vi "Find by Path Test.vi"() -> ()   [LabVIEW 2017]
uses:
  String Subset.vi
  Offset/Find Item Locations by Path.vi
  Parsing/Parse Full Path or Item Name.vi
  <vilib>/addons/_JKI Toolkits/Caraya/classes/Test/Test.lvclass
  <vilib>/addons/_JKI Toolkits/Caraya/classes/Assert/Assert.lvclass
  JSONtext.lvlib
panel:
  out "error out":errorcluster
  out "Path":string[](array[string])
  out "Time (s)":dbl[](array[numeric]) format="%#_3p"
  out "Array":string[](array[string])
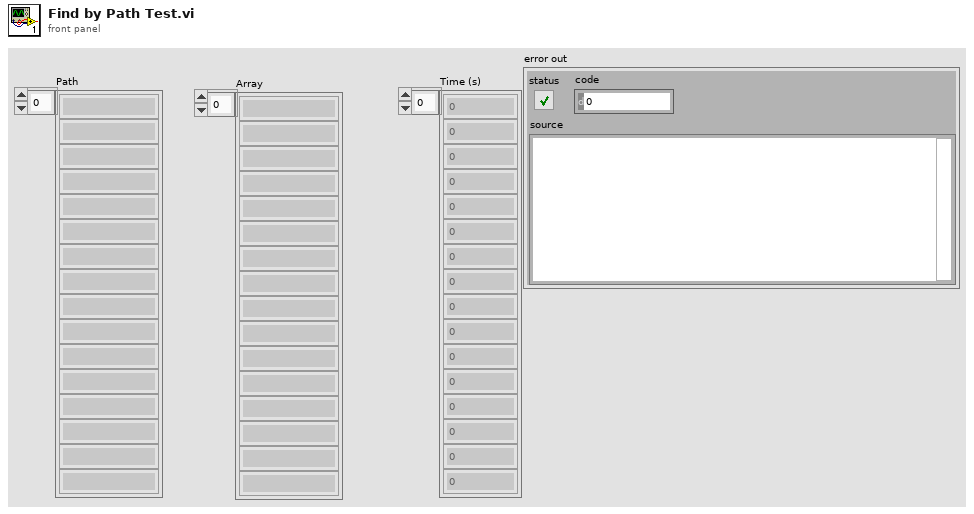
[diagram p1: front panel]
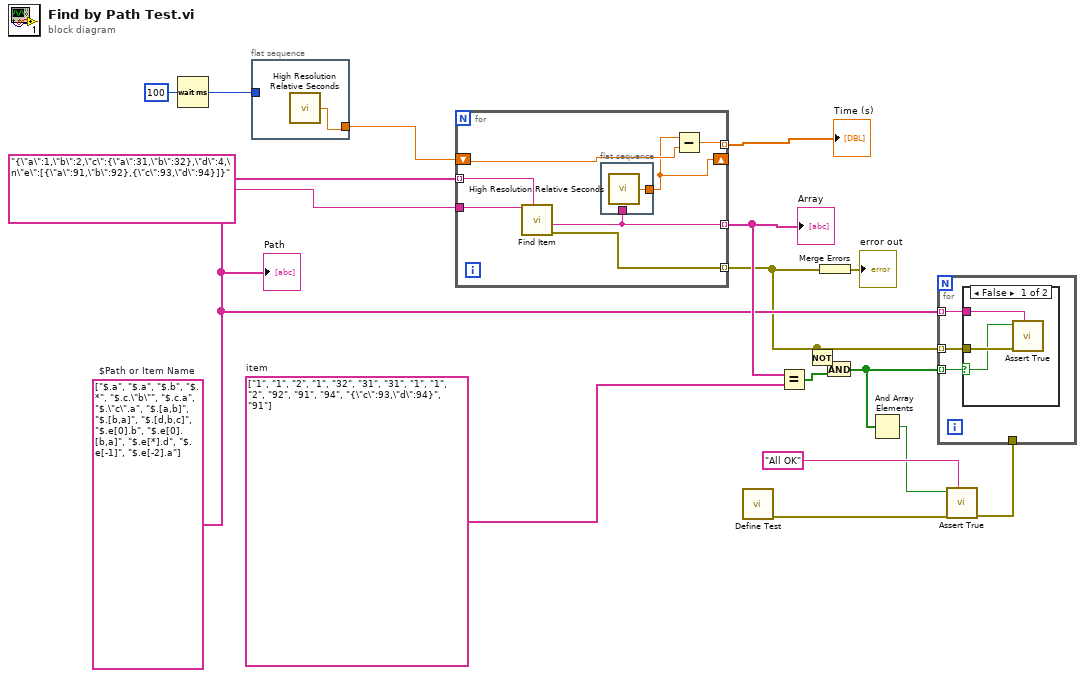
[diagram p0: block diagram]
diagram:
  w8 = string[] ["1", "1", "2", "1", "32", "31", "31", "1", "1", "2", "92", "91", "94", "{\"c\":93,\"d\":94}", "91"]  # item
  w3 = string[] ["$.a", "$.a", "$.b", "$.*", "$.c.\"b\"", "$.c.a", "$.\"c\".a", "$.[a,b]", "$.[b,a]", "$.[d,b,c]", "$.e[0].b", "$.e[0].[b,a]", "$.e[*].d", "$.e[-1]", "$.e[-2].a"]  # $Path or Item Name
  n1 = Wait (ms)(milliseconds to wait=u32 100) -> (millisecond timer value=w6:u32)
  n2 = flat-sequence {
    tunnel: [w18] -> w5
    tunnel: w6 -> [_]
    frame #0 {
      n3 = call <vilib>:"High Resolution Relative Seconds.vi"() -> ("relative seconds"=w18:dbl)
    }
  }
  n4 = for {
    tunnel: "{\"a\":1,\"b\":2,\"c\":{\"a\":31,\"b\":32},\"d\":4,\n\"e\":[{\"a\":91,\"b\":92},{\"c\":93,\"d\":94}]}" -> [w25]
    tunnel: w3 -> [w24] mode=indexing
    tunnel: [w22] -> w14 mode=indexing
    tunnel: [w23] -> w2 mode=indexing
    shift-right: [w20] -> _
    shift-left: w5 -> [w21]
    tunnel: [w19] -> w4 mode=indexing
    n5 = call "Find Item.vi"("$Path or Item Name"=w24, "JSON"=w25) -> ("error out"=w23:errorcluster, "<JSON>"=w22:string)  [unwired: 6 in, 2 out]
    n6 = flat-sequence {
      tunnel: [w26] -> w20
      tunnel: w22 -> [_]
      frame #0 {
        n7 = call <vilib>:"High Resolution Relative Seconds.vi"() -> ("relative seconds"=w26:dbl)
      }
    }
    n8 = Subtract(x=w20, y=w21) -> (x-y=w19:dbl)
  }
  "Array" <- w14
  "Time (s)" <- w4
  n9 = call <vilib>:"Define Test.vi"() -> ("error out"=w16:errorcluster)  [unwired: 11 in]
  n10 = Equal?(x=w14, y=w8) -> (x = y?=w13:bool[])
  n11 = Not(x=w2) -> (.not. x?=w12:bool[])
  n12 = Merge Errors(w2) -> (→"error out":errorcluster)
  n13 = And(x=w12, y=w13) -> (x .and. y?=w11:bool[])
  n14 = And Array Elements(Boolean array=w11) -> (logical AND=w10:bool)
  n15 = call <vilib>:"Assert True.vi"("Label"="All OK", "error in (no error)"=w16, "True?"=w10) -> ("error out"=w9:errorcluster)  [unwired: 8 in]
  n16 = for {
    tunnel: w3 -> [w29] mode=indexing
    tunnel: w2 -> [w28] mode=indexing
    tunnel: w11 -> [w27] mode=indexing
    tunnel: w9 -> [_]
    n17 = case shown="False" w27 {
      selector: w27 -> [w30 _]
      tunnel: w29 -> [w32 _]
      tunnel: w28 -> [w31 _]
      frame False {
        n18 = call <vilib>:"Assert True.vi"("Label"=w32, "error in (no error)"=w31, "True?"=w30) -> ()  [unwired: 8 in, 1 out]
      }
      frame True {
      }
    }
  }
  "Path" <- w3
